vi "GetHelp.vi"(11 "MassCompile in":refnum<class "MassCompile.lvclass">) -> (2 "Help":string, 3 "MassCompile out":refnum<class "MassCompile.lvclass">)   [LabVIEW 2014, in "MassCompile.lvclass"]
uses:
  MassCompile.lvclass
panel:
  in  "Help":string="LabVIEWCLI -OperationName MassCompile -DirectoryToCompile <path of directory to mass compile>  [-MassCompileLogFile <mass compile log file path>]  [-AppendToMassCompileLog <TRUE or FALSE>]  [-NumberOfVIsToCache <numeric value>]  [-ReloadLVSBs <true or false>]\n\n -DirectoryToCompile : Specifies the directory where the mass compile should begin. This is required argument.\n -MassCompileLogFile : Specifies a file path where results of the mass compile should be placed. Default value is No file.\n -AppendToMassCompileLog : Specifies whether results should be appended to the log file. Default value is FALSE.\n -NumberOfVIsToCache : Specifies the number of VIs that should be allowed to remain in memory during the mass compile. Default value is 0.\n -ReloadLVSBs : If TRUE, causes CINs in VIs to be ignored and the application to search for them. Useful when a large number of CINs have been recompiled and need to be reloaded. Default value is FALSE."
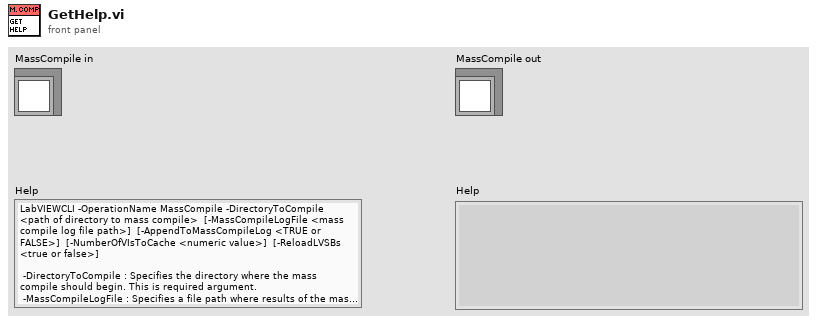
[diagram p1: front panel]
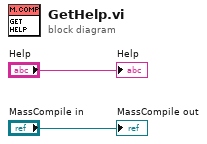
[diagram p0: block diagram]
diagram:
  "MassCompile out" <- "MassCompile in"
  "Help" <- "Help"
